vi "OE1311&OE1351_DATA Transmit.vi"(0 "Input Data":u8[](array[numeric])) -> (1 "Total Date Array":dbl[][](array[numeric]), 2 "Parameter Values":T2, 3 "PLL&Overload":T1, 4 "Trig_Count":u8[](array[numeric]))   [LabVIEW 2011]
panel:
  out "Xita h7":dbl[](array[numeric])
  out "Xh7":dbl[](array[numeric])
  out "Rh7":dbl[](array[numeric])
  out "Yh7":dbl[](array[numeric])
  out "Xita h6":dbl[](array[numeric])
  out "Rh4":dbl[](array[numeric])
  out "Xh4":dbl[](array[numeric])
  out "Xita h4":dbl[](array[numeric])
  out "Xh5":dbl[](array[numeric])
  out "Xita h5":dbl[](array[numeric])
  out "Xh6":dbl[](array[numeric])
  out "Yh4":dbl[](array[numeric])
  out "Yh5":dbl[](array[numeric])
  out "Rh5":dbl[](array[numeric])
  out "Yh6":dbl[](array[numeric])
  out "Rh6":dbl[](array[numeric])
  out "X":dbl[](array[numeric])
  out "Y":dbl[](array[numeric])
  out "Frequency":dbl[](array[numeric])
  out "XNoise":dbl[](array[numeric])
  out "Xh1":dbl[](array[numeric])
  out "Yh1":dbl[](array[numeric])
  out "Xh2":dbl[](array[numeric])
  out "Yh2":dbl[](array[numeric])
  out "AUXADC1":dbl[](array[numeric])
  out "AUXADC2":dbl[](array[numeric])
  out "Xh3":dbl[](array[numeric])
  out "Yh3":dbl[](array[numeric])
  out "YNoise":dbl[](array[numeric])
  out "R":dbl[](array[numeric])
  out "Xita":dbl[](array[numeric])
  out "Rh1":dbl[](array[numeric])
  out "Xita h1":dbl[](array[numeric])
  out "Rh2":dbl[](array[numeric])
  out "Xitah2":dbl[](array[numeric])
  out "Rh3":dbl[](array[numeric])
  out "Xita h3":dbl[](array[numeric])
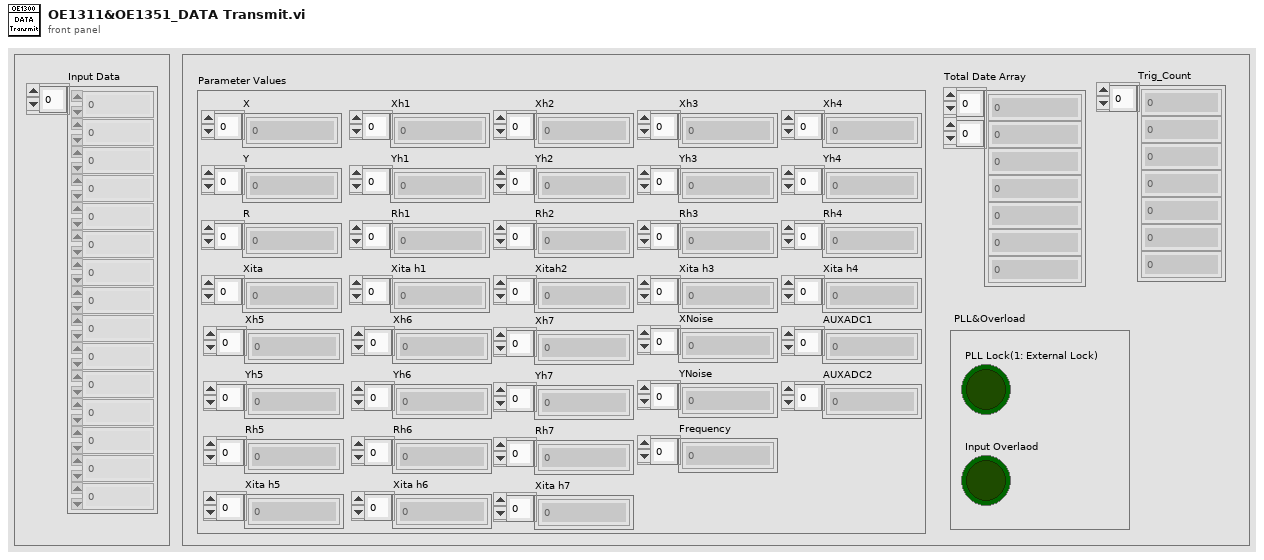
[diagram p1: front panel]
types:
  T1 = cluster{"PLL Lock(1: External Lock)":bool, "Input Overlaod":bool}
  T2 = cluster{"X":dbl[], "Y":dbl[], "R":dbl[], "Xita":dbl[], "XNoise":dbl[], "YNoise":dbl[], "Frequency":dbl[], "Xh1":dbl[], "Yh1":dbl[], "Rh1":dbl[], "Xita h1":dbl[], "Xh2":dbl[], "Yh2":dbl[], "Rh2":dbl[], "Xitah2":dbl[], "Xh3":dbl[], "Yh3":dbl[], "Rh3":dbl[], "Xita h3":dbl[], "Xh4":dbl[], "Yh4":dbl[], "Rh4":dbl[], "Xita h4":dbl[], "Xh5":dbl[], "Yh5":dbl[], "Rh5":dbl[], "Xita h5":dbl[], "Xh6":dbl[], "Yh6":dbl[], "Rh6":dbl[], "Xita h6":dbl[], "Xh7":dbl[], "Yh7":dbl[], "Rh7":dbl[], "Xita h7":dbl[], "AUXADC1":dbl[], "AUXADC2":dbl[]}
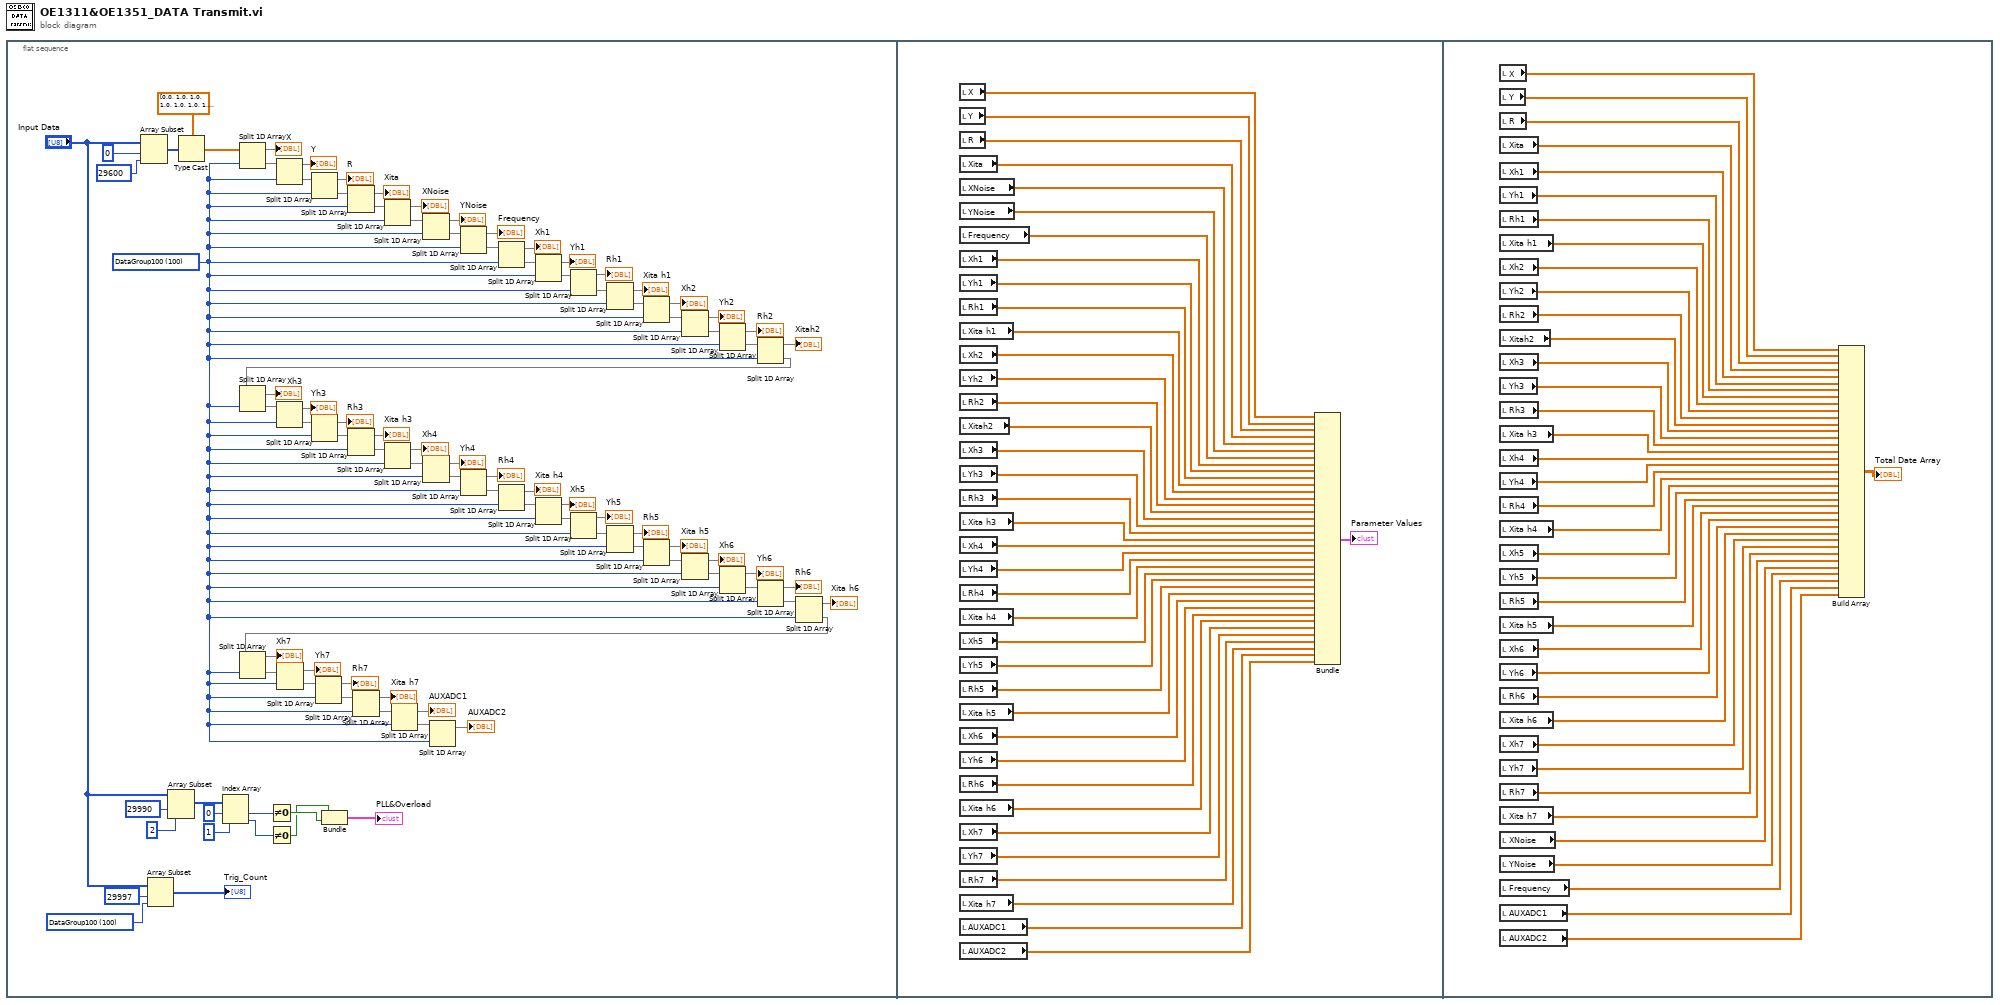
[diagram p0: block diagram]
diagram:
  n1 = flat-sequence {
    frame #0 {
      w4 = u16 100 items=["unsignedInt8"=1, "unsignedInt16"=2, "unsignedInt32"=4, "unsignedInt64"=8, "Float"=80, "Double"=160, "StartLength"=2240, "DataGroup50"=50, "DataGroup100"=100, "DataGroup20"=20] ("数据类型")
      w15 = u16 100 items=["unsignedInt8"=1, "unsignedInt16"=2, "unsignedInt32"=4, "unsignedInt64"=8, "Float"=80, "Double"=160, "StartLength"=2240, "DataGroup50"=50, "DataGroup100"=100, "DataGroup20"=20] ("数据类型")
      n2 = Array Subset(array="Input Data", index=0 ("索引"), length=29600 ("长度")) -> (w91:u8[])
      n3 = Array Subset(array="Input Data", index=29997 ("索引"), length=w4) -> (→"Trig_Count":u8[])
      n4 = Array Subset(array="Input Data", index=29990 ("索引"), length=2 ("长度")) -> (w12:u8[])
      n5 = Type Cast(type=dbl[] [0.0, 1.0, 1.0, 1.0, 1.0, 1.0, 1.0, 1.0, 1.0, 1.0, 1.0, 1.0, 1.0, 1.0, 1.0, 1.0, 1.0, 1.0, 1.0, 1.0, 1.0, 1.0, 1.0, 1.0, 1.0, 1.0, 1.0, 1.0, 1.0, 1.0, 1.0, 1.0, 1.0, 1.0, 1.0, 1.0, 1.0, 1.0, 1.0, 1.0, 1.0, 1.0, 1.0, 1.0, 1.0, 1.0, 1.0, 1.0, 1.0, 1.0, 1.0, 1.0, 1.0, 1.0, 1.0, 1.0, 1.0, 1.0, 1.0, 1.0, 1.0, 1.0, 1.0, 1.0, 1.0, 1.0, 1.0, 1.0, 1.0, 1.0, 1.0, 1.0, 1.0, 1.0, 1.0, 1.0, 1.0, 1.0, 1.0, 1.0, 1.0, 1.0, 1.0, 1.0, 1.0, 1.0, 1.0, 1.0, 1.0, 1.0, 1.0, 1.0, 1.0, 1.0, 1.0, 1.0, 1.0, 1.0, 1.0, 1.0, 1.0, 1.0, 1.0, 1.0, 1.0, 1.0, 1.0, 1.0, 1.0, 1.0, 1.0, 1.0, 1.0, 1.0, 1.0, 1.0, 1.0, 1.0, 1.0, 1.0, 1.0, 1.0, 1.0, 1.0, 1.0, 1.0, 1.0, 1.0, 1.0, 1.0, 1.0, 1.0, 1.0, 1.0, 1.0, 1.0, 1.0, 1.0, 1.0, 1.0, 1.0, 1.0, 1.0, 1.0, 1.0, 1.0, 1.0, 1.0, 1.0, 1.0, 1.0, 1.0, 1.0, 1.0, 1.0, 1.0, 1.0, 1.0, 1.0, 1.0, 1.0, 1.0, 1.0, 1.0, 1.0, 1.0, 1.0, 1.0, 1.0, 1.0, 1.0, 1.0, 1.0, 1.0, 1.0, 1.0, 1.0, 1.0, 1.0, 1.0, 1.0, 1.0, 1.0, 1.0, 1.0, 1.0, 1.0, 1.0, 1.0, 1.0, 1.0, 1.0, 1.0, 1.0, 1.0, 1.0, 1.0, 1.0, 1.0, 1.0, 1.0, 1.0, 1.0, 1.0, 1.0, 1.0, 1.0, 1.0, 1.0, 1.0, 1.0, 1.0, 1.0, 1.0, 1.0, 1.0, 1.0, 1.0, 1.0, 1.0, 1.0, 1.0, 1.0, 1.0, 1.0, 1.0, 1.0, 1.0, 1.0, 1.0, 1.0, 1.0, 1.0, 1.0, 1.0, 1.0, 1.0, 1.0, 1.0, 1.0, 1.0, 1.0, 1.0, 1.0, 1.0, 1.0, 1.0, 1.0, 1.0, 1.0, 1.0, 1.0, 1.0, 1.0, 1.0, 1.0, 1.0, 1.0, 1.0, 1.0, 1.0, 1.0, 1.0, 1.0, 1.0, 1.0, 1.0, 1.0, 1.0, 1.0, 1.0, 1.0, 1.0, 1.0, 1.0, 1.0, 1.0, 1.0, 1.0, 1.0, 1.0, 1.0, 1.0, 1.0, 1.0, 1.0, 1.0, 1.0, 1.0, 1.0, 1.0, 1.0, 1.0, 1.0, 1.0, 1.0, 1.0, 1.0, 1.0, 1.0, 1.0, 1.0, 1.0, 1.0, 1.0, 1.0, 1.0, 1.0, 1.0, 1.0, 1.0, 1.0, 1.0, 1.0, 1.0, 1.0, 1.0, 1.0, 1.0, 1.0, 1.0, 1.0, 1.0, 1.0, 1.0, 1.0, 1.0, 1.0, 1.0, 1.0, 1.0, 1.0, 1.0, 1.0, 1.0, 1.0, 1.0, 1.0, 1.0, 1.0, 1.0, 1.0, 1.0, 1.0, 1.0, 1.0, 1.0, 1.0, 1.0, 1.0, 1.0, 1.0, 1.0, 1.0, 1.0, 1.0, 1.0, 1.0, 1.0, 1.0, 1.0, 1.0, 1.0, 1.0, 1.0, 1.0, 1.0, 1.0, 1.0, 1.0, 1.0, 1.0, 1.0, 1.0, 1.0, 1.0, 1.0, 1.0, 1.0, 1.0, 1.0, 1.0, 1.0, 1.0, 1.0, 1.0, 1.0, 1.0, 1.0, 1.0, 1.0, 1.0, 1.0, 1.0, 1.0, 1.0, 1.0, 1.0, 1.0, 1.0, 0.0, 1.0, 1.0, 1.0, 1.0, 1.0, 1.0, 1.0, 1.0, 1.0, 1.0, 1.0, 1.0, 1.0, 1.0, 1.0, 1.0, 1.0, 1.0, 1.0, 1.0, 1.0, 1.0, 1.0, 1.0, 1.0, 1.0, 1.0, 1.0, 1.0, 1.0, 1.0, 1.0, 1.0, 1.0, 1.0, 1.0, 1.0, 1.0, 1.0, 1.0, 1.0, 1.0, 1.0, 1.0, 1.0, 1.0, 1.0, 1.0, 1.0, 1.0, 1.0, 1.0, 1.0, 1.0, 1.0, 1.0, 1.0, 1.0, 1.0, 1.0, 1.0, 1.0, 1.0, 1.0, 1.0, 1.0, 1.0, 1.0, 1.0, 1.0, 1.0, 1.0, 1.0, 1.0, 1.0, 1.0, 1.0, 1.0, 1.0, 1.0, 1.0, 1.0, 1.0, 1.0, 1.0, 1.0, 1.0, 1.0, 1.0, 1.0, 1.0, 1.0, 1.0, 1.0, 1.0, 1.0, 1.0, 1.0, 1.0, 1.0, 1.0, 1.0, 1.0, 1.0, 1.0, 1.0, 1.0, 1.0, 1.0, 1.0, 1.0, 1.0, 1.0, 1.0, 1.0, 1.0, 1.0, 1.0, 1.0, 1.0, 1.0, 1.0, 1.0, 1.0, 1.0, 1.0, 1.0, 1.0, 1.0, 1.0, 1.0, 1.0, 1.0, 1.0, 1.0, 1.0, 1.0, 1.0, 1.0, 1.0, 1.0, 1.0, 1.0, 1.0, 1.0, 1.0, 1.0, 1.0, 1.0, 1.0, 1.0, 1.0, 1.0, 1.0, 1.0, 1.0, 1.0, 1.0, 1.0, 1.0, 1.0, 1.0, 1.0, 1.0, 1.0, 1.0, 1.0, 1.0, 1.0, 1.0, 1.0, 1.0, 1.0, 1.0, 1.0, 1.0, 1.0, 1.0, 1.0, 1.0, 1.0, 1.0, 1.0, 1.0, 1.0, 1.0, 1.0, 1.0, 1.0, 1.0, 1.0, 1.0, 1.0, 1.0, 1.0, 1.0, 1.0, 1.0, 1.0, 1.0, 1.0, 1.0, 1.0, 1.0, 1.0, 1.0, 1.0, 1.0, 1.0, 1.0, 1.0, 1.0, 1.0, 1.0, 1.0, 1.0, 1.0, 1.0, 1.0, 1.0, 1.0, 1.0, 1.0, 1.0, 1.0, 1.0, 1.0, 1.0, 1.0, 1.0, 1.0, 1.0, 1.0, 1.0, 1.0, 1.0, 1.0, 1.0, 1.0, 1.0, 1.0, 1.0, 1.0, 1.0, 1.0, 1.0, 1.0, 1.0, 1.0, 1.0, 1.0, 1.0, 1.0, 1.0, 1.0, 1.0, 1.0, 1.0, 1.0, 1.0, 1.0, 1.0, 1.0, 1.0, 1.0, 1.0, 1.0, 1.0, 1.0, 1.0, 1.0, 1.0, 1.0, 1.0, 1.0, 1.0, 1.0, 1.0, 1.0, 1.0, 1.0, 1.0, 1.0, 1.0, 1.0, 1.0, 1.0, 1.0, 1.0, 1.0, 1.0, 1.0, 1.0, 1.0, 1.0, 1.0, 1.0, 1.0, 1.0, 1.0, 1.0, 1.0, 1.0, 1.0, 1.0, 1.0, 1.0, 1.0, 1.0, 1.0, 1.0, 1.0, 1.0, 1.0, 1.0, 1.0, 1.0, 1.0, 1.0, 1.0, 1.0, 1.0, 1.0, 1.0, 1.0, 1.0, 1.0, 1.0, 1.0, 1.0, 1.0, 1.0, 1.0, 1.0, 1.0, 1.0, 1.0, 1.0, 1.0, 1.0, 1.0, 1.0, 1.0, 1.0, 1.0, 1.0, 1.0, 1.0, 1.0, 1.0, 1.0, 1.0, 1.0, 1.0, 1.0, 1.0, 1.0, 1.0, 1.0, 1.0, 1.0, 1.0, 1.0, 1.0, 1.0, 1.0, 1.0, 1.0, 1.0, 1.0, 1.0, 1.0, 1.0, 1.0, 1.0, 1.0, 1.0, 1.0, 1.0, 1.0, 1.0, 1.0, 1.0, 1.0, 1.0, 1.0, 1.0, 1.0, 1.0, 1.0, 1.0, 1.0, 1.0, 1.0, 1.0, 1.0, 1.0, 1.0, 1.0], x=w91) -> (*(type *) &x=w89:dbl[])
      n6 = Index Array(array=w12, index #1=0 ("索引"), index #2=1 ("索引")) -> (element #1=w9:u8, element #2=w8:u8)
      n7 = Split 1D Array(array=w89, index=w15) -> (first subarray=→"X":dbl[], second subarray=w90:dbl[])
      n8 = Not Equal To 0?(x=w9) -> (x != 0?=w2:bool)
      n9 = Not Equal To 0?(x=w8) -> (x != 0?=w1:bool)
      n10 = Split 1D Array(array=w90, index=w15) -> (first subarray=→"Y":dbl[], second subarray=w92:dbl[])
      n11 = Split 1D Array(array=w92, index=w15) -> (first subarray=→"R":dbl[], second subarray=w82:dbl[])
      n12 = Bundle(w1, w2) -> (→"PLL&Overload":cluster{bool, bool})  [unwired: 1 in]
      n13 = Split 1D Array(array=w82, index=w15) -> (first subarray=→"Xita":dbl[], second subarray=w84:dbl[])
      n14 = Split 1D Array(array=w84, index=w15) -> (first subarray=→"XNoise":dbl[], second subarray=w83:dbl[])
      n15 = Split 1D Array(array=w83, index=w15) -> (first subarray=→"YNoise":dbl[], second subarray=w76:dbl[])
      n16 = Split 1D Array(array=w76, index=w15) -> (first subarray=→"Frequency":dbl[], second subarray=w74:dbl[])
      n17 = Split 1D Array(array=w74, index=w15) -> (first subarray=→"Xh1":dbl[], second subarray=w73:dbl[])
      n18 = Split 1D Array(array=w73, index=w15) -> (first subarray=→"Yh1":dbl[], second subarray=w72:dbl[])
      n19 = Split 1D Array(array=w72, index=w15) -> (first subarray=→"Rh1":dbl[], second subarray=w68:dbl[])
      n20 = Split 1D Array(array=w68, index=w15) -> (first subarray=→"Xita h1":dbl[], second subarray=w66:dbl[])
      n21 = Split 1D Array(array=w66, index=w15) -> (first subarray=→"Xh2":dbl[], second subarray=w64:dbl[])
      n22 = Split 1D Array(array=w64, index=w15) -> (first subarray=→"Yh2":dbl[], second subarray=w93:dbl[])
      n23 = Split 1D Array(array=w93, index=w15) -> (first subarray=→"Rh2":dbl[], second subarray=w85:dbl[])
      n24 = Split 1D Array(array=w85, index=w15) -> (first subarray=→"Xitah2":dbl[], second subarray=w34:dbl[])
      n25 = Split 1D Array(array=w34, index=w15) -> (first subarray=→"Xh3":dbl[], second subarray=w37:dbl[])
      n26 = Split 1D Array(array=w37, index=w15) -> (first subarray=→"Yh3":dbl[], second subarray=w36:dbl[])
      n27 = Split 1D Array(array=w36, index=w15) -> (first subarray=→"Rh3":dbl[], second subarray=w41:dbl[])
      n28 = Split 1D Array(array=w41, index=w15) -> (first subarray=→"Xita h3":dbl[], second subarray=w39:dbl[])
      n29 = Split 1D Array(array=w39, index=w15) -> (first subarray=→"Xh4":dbl[], second subarray=w40:dbl[])
      n30 = Split 1D Array(array=w40, index=w15) -> (first subarray=→"Yh4":dbl[], second subarray=w43:dbl[])
      n31 = Split 1D Array(array=w43, index=w15) -> (first subarray=→"Rh4":dbl[], second subarray=w45:dbl[])
      n32 = Split 1D Array(array=w45, index=w15) -> (first subarray=→"Xita h4":dbl[], second subarray=w46:dbl[])
      n33 = Split 1D Array(array=w46, index=w15) -> (first subarray=→"Xh5":dbl[], second subarray=w47:dbl[])
      n34 = Split 1D Array(array=w47, index=w15) -> (first subarray=→"Yh5":dbl[], second subarray=w51:dbl[])
      n35 = Split 1D Array(array=w51, index=w15) -> (first subarray=→"Rh5":dbl[], second subarray=w53:dbl[])
      n36 = Split 1D Array(array=w53, index=w15) -> (first subarray=→"Xita h5":dbl[], second subarray=w55:dbl[])
      n37 = Split 1D Array(array=w55, index=w15) -> (first subarray=→"Xh6":dbl[], second subarray=w35:dbl[])
      n38 = Split 1D Array(array=w35, index=w15) -> (first subarray=→"Yh6":dbl[], second subarray=w38:dbl[])
      n39 = Split 1D Array(array=w38, index=w15) -> (first subarray=→"Rh6":dbl[], second subarray=w29:dbl[])
      n40 = Split 1D Array(array=w29, index=w15) -> (first subarray=→"Xita h6":dbl[], second subarray=w16:dbl[])
      n41 = Split 1D Array(array=w16, index=w15) -> (first subarray=→"Xh7":dbl[], second subarray=w18:dbl[])
      n42 = Split 1D Array(array=w18, index=w15) -> (first subarray=→"Yh7":dbl[], second subarray=w24:dbl[])
      n43 = Split 1D Array(array=w24, index=w15) -> (first subarray=→"Rh7":dbl[], second subarray=w22:dbl[])
      n44 = Split 1D Array(array=w22, index=w15) -> (first subarray=→"Xita h7":dbl[], second subarray=w23:dbl[])
      n45 = Split 1D Array(array=w23, index=w15) -> (first subarray=→"AUXADC1":dbl[], second subarray=w21:dbl[])
      n46 = Split 1D Array(array=w21, index=w15) -> (first subarray=→"AUXADC2":dbl[])  [unwired: 1 out]
    }
    frame #1 {
      n47 = local read "X"() -> (w131:dbl[])
      n48 = local read "Y"() -> (w130:dbl[])
      n49 = local read "R"() -> (w129:dbl[])
      n50 = local read "Xita"() -> (w128:dbl[])
      n51 = local read "XNoise"() -> (w127:dbl[])
      n52 = local read "YNoise"() -> (w126:dbl[])
      n53 = local read "Frequency"() -> (w125:dbl[])
      n54 = local read "Xh1"() -> (w124:dbl[])
      n55 = local read "Yh1"() -> (w123:dbl[])
      n56 = local read "Rh1"() -> (w122:dbl[])
      n57 = local read "Xita h1"() -> (w121:dbl[])
      n58 = local read "Xh2"() -> (w120:dbl[])
      n59 = local read "Yh2"() -> (w119:dbl[])
      n60 = local read "Rh2"() -> (w118:dbl[])
      n61 = local read "Xitah2"() -> (w117:dbl[])
      n62 = local read "Xh3"() -> (w98:dbl[])
      n63 = local read "Yh3"() -> (w97:dbl[])
      n64 = local read "Rh3"() -> (w96:dbl[])
      n65 = local read "Xita h3"() -> (w95:dbl[])
      n66 = local read "Xh4"() -> (w116:dbl[])
      n67 = local read "Yh4"() -> (w115:dbl[])
      n68 = local read "Rh4"() -> (w114:dbl[])
      n69 = local read "Xita h4"() -> (w113:dbl[])
      n70 = local read "Xh5"() -> (w112:dbl[])
      n71 = local read "Yh5"() -> (w111:dbl[])
      n72 = local read "Rh5"() -> (w110:dbl[])
      n73 = local read "Xita h5"() -> (w109:dbl[])
      n74 = local read "Xh6"() -> (w108:dbl[])
      n75 = local read "Yh6"() -> (w107:dbl[])
      n76 = local read "Rh6"() -> (w106:dbl[])
      n77 = local read "Xita h6"() -> (w105:dbl[])
      n78 = local read "Xh7"() -> (w104:dbl[])
      n79 = local read "Yh7"() -> (w103:dbl[])
      n80 = local read "Rh7"() -> (w102:dbl[])
      n81 = local read "Xita h7"() -> (w101:dbl[])
      n82 = local read "AUXADC1"() -> (w100:dbl[])
      n83 = local read "AUXADC2"() -> (w99:dbl[])
      n84 = Bundle("X"=w131, "Y"=w130, "R"=w129, "Xita"=w128, "XNoise"=w127, "YNoise"=w126, "Frequency"=w125, "Xh1"=w124, "Yh1"=w123, "Rh1"=w122, "Xita h1"=w121, "Xh2"=w120, "Yh2"=w119, "Rh2"=w118, "Xitah2"=w117, "Xh3"=w98, "Yh3"=w97, "Rh3"=w96, "Xita h3"=w95, "Xh4"=w116, "Yh4"=w115, "Rh4"=w114, "Xita h4"=w113, "Xh5"=w112, "Yh5"=w111, "Rh5"=w110, "Xita h5"=w109, "Xh6"=w108, "Yh6"=w107, "Rh6"=w106, "Xita h6"=w105, "Xh7"=w104, "Yh7"=w103, "Rh7"=w102, "Xita h7"=w101, "AUXADC1"=w100, "AUXADC2"=w99) -> (→"Parameter Values":T2)  [unwired: 1 in]
    }
    frame #2 {
      n85 = local read "X"() -> (w169:dbl[])
      n86 = local read "Y"() -> (w168:dbl[])
      n87 = local read "R"() -> (w167:dbl[])
      n88 = local read "Xita"() -> (w166:dbl[])
      n89 = local read "Xh1"() -> (w165:dbl[])
      n90 = local read "Yh1"() -> (w164:dbl[])
      n91 = local read "Rh1"() -> (w163:dbl[])
      n92 = local read "Xita h1"() -> (w162:dbl[])
      n93 = local read "Xh2"() -> (w161:dbl[])
      n94 = local read "Yh2"() -> (w160:dbl[])
      n95 = local read "Rh2"() -> (w159:dbl[])
      n96 = local read "Xitah2"() -> (w158:dbl[])
      n97 = local read "Xh3"() -> (w139:dbl[])
      n98 = local read "Yh3"() -> (w138:dbl[])
      n99 = local read "Rh3"() -> (w137:dbl[])
      n100 = local read "Xita h3"() -> (w136:dbl[])
      n101 = local read "Xh4"() -> (w157:dbl[])
      n102 = local read "Yh4"() -> (w156:dbl[])
      n103 = local read "Rh4"() -> (w155:dbl[])
      n104 = local read "Xita h4"() -> (w154:dbl[])
      n105 = local read "Xh5"() -> (w153:dbl[])
      n106 = local read "Yh5"() -> (w152:dbl[])
      n107 = local read "Rh5"() -> (w151:dbl[])
      n108 = local read "Xita h5"() -> (w150:dbl[])
      n109 = local read "Xh6"() -> (w149:dbl[])
      n110 = local read "Yh6"() -> (w148:dbl[])
      n111 = local read "Rh6"() -> (w147:dbl[])
      n112 = local read "Xita h6"() -> (w146:dbl[])
      n113 = local read "Xh7"() -> (w145:dbl[])
      n114 = local read "Yh7"() -> (w144:dbl[])
      n115 = local read "Rh7"() -> (w143:dbl[])
      n116 = local read "Xita h7"() -> (w142:dbl[])
      n117 = local read "XNoise"() -> (w135:dbl[])
      n118 = local read "YNoise"() -> (w134:dbl[])
      n119 = local read "Frequency"() -> (w133:dbl[])
      n120 = local read "AUXADC1"() -> (w141:dbl[])
      n121 = local read "AUXADC2"() -> (w140:dbl[])
      n122 = Build Array(w169, w168, w167, w166, w165, w164, w163, w162, w161, w160, w159, w158, w139, w138, w137, w136, w157, w156, w155, w154, w153, w152, w151, w150, w149, w148, w147, w146, w145, w144, w143, w142, w135, w134, w133, w141, w140) -> (→"Total Date Array":dbl[][])
    }
  }
